vi "自由间隙.vi"(0 "曲线引用":refnum<vi>, 1 "自由间隙判定条件":cluster{"下限":dbl, "上限":dbl}, 3 "错误输入":errorcluster) -> (7 "曲线引用输出":refnum<vi>, 8 "OK？":bool, 10 "错误输出":errorcluster)   [LabVIEW 2018]
uses:
  Global_Variable/Global.vi
  Global_Variable/A180648.vi
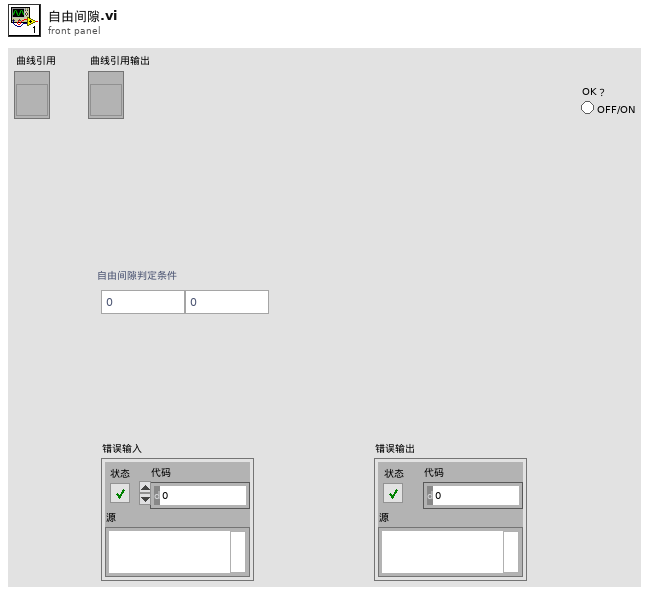
[diagram p1: front panel]
types:
  T1 = enum32{"空载", "功能", "力特性", "传感器特性", "电流特性", "振动NVH", "逆向空载", "完成"}
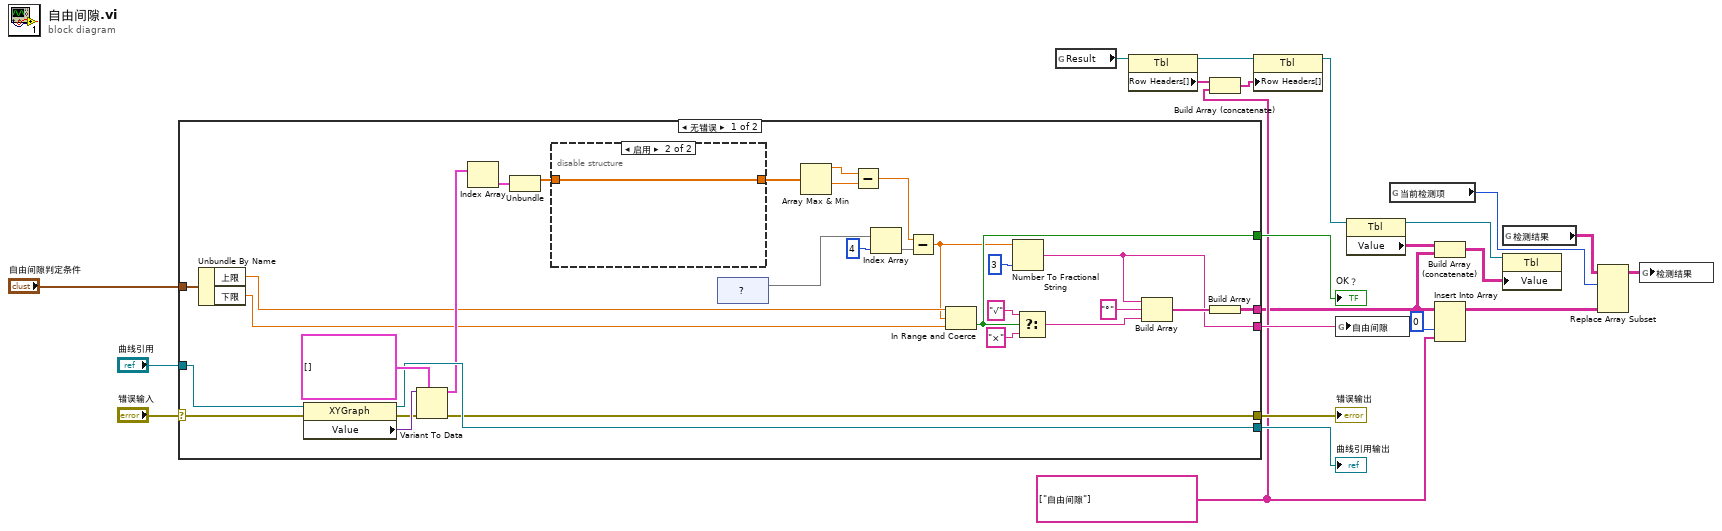
[diagram p0: block diagram]
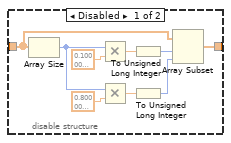
[diagram p2: hidden frame]
diagram:
  w7 = string[] ["自由间隙"] ("列首字符串[]")
  n1 = case shown="无错误" "错误输入" {
    selector: "错误输入" -> [w50 w64]
    tunnel: [w47 w64] -> w21
    tunnel: "曲线引用" -> [w46 w63]
    tunnel: [w49 w63] -> w19
    tunnel: [w33 _] -> w18
    tunnel: "自由间隙判定条件" -> [w36 _]
    tunnel: [w37 _] -> w1
    tunnel: [w25 _] -> w9
    frame No Error {
      n2 = Unbundle By Name(w36) -> ("上限"=w35:dbl, "下限"=w34:dbl)
      n3 = property class="XYGraph"(reference=w46, error in=w50) -> (reference out=w49:refnum<vi>, error out=w48:errorcluster, "Value"=w52:variant)
      n4 = Variant To Data(error in=w48, type=cluster{dbl[], dbl[]}[] [], Variant=w52) -> (data=w40:cluster{dbl[], dbl[]}[], error out=w47:errorcluster)
      n5 = Index Array(array=w40) -> (element=w39:cluster{dbl[], dbl[]})  [unwired: 1 in]
      n6 = Unbundle(w39) -> (w24:dbl[])  [unwired: 1 out]
      n7 = disable-structure shown="启用" {
        disable-tunnel: w24 -> [w54 w62]
        disable-tunnel: [w53 w62] -> w23
        frame Disabled {
          n8 = Array Size(array=w54) -> (size(s)=w57:i32)
          n9 = Multiply(x=w57, y=sgl 0.1) -> (x*y=w59:sgl)
          n10 = Multiply(x=w57, y=sgl 0.8) -> (x*y=w60:sgl)
          n11 = To Unsigned Long Integer(number=w59) -> (unsigned 32bit integer=w61:u32)
          n12 = To Unsigned Long Integer(number=w60) -> (unsigned 32bit integer=w58:u32)
          n13 = Array Subset(array=w54, index=w61, length=w58) -> (w53:dbl[])
        }
        frame Enabled {
        }
      }
      n14 = shared-variable "?"() -> (w29)  [unwired: 1 in, 1 out]
      n15 = Array Max & Min(array=w23) -> (max value=w32:dbl, min value=w31:dbl)  [unwired: 2 out]
      n16 = Subtract(x=w32, y=w31) -> (x-y=w30:dbl)
      n17 = Index Array(array=w29, index=4 ("索引")) -> (element=w27)
      n18 = Subtract(x=w30, y=w27) -> (x-y=w26:dbl)
      n19 = In Range and Coerce(upper limit=w35, x=w26, lower limit=w34) -> (In Range?=w33:bool)  [unwired: 1 out]
      n20 = Number To Fractional String(number=w26, precision (6)=i16 3 ("精度(6)")) -> (F-format string=w25:string)  [unwired: 2 in]
      n21 = Select(t="√" ("元素"), s=w33, f="×" ("元素")) -> (s? t:f=w41:string)
      n22 = Build Array(w25, "°" ("元素"), w41) -> (w38:string[])
      n23 = Build Array(w38) -> (w37:string[][])
    }
    frame Error {
    }
  }
  "错误输出" <- w21
  "曲线引用输出" <- w19
  "OK？" <- w18
  n24 = global read "Global.vi" "Result"() -> (w15:refnum<vi>)
  n25 = property class="Tbl"(reference=w15) -> (reference out=w14:refnum<vi>, "Row Headers[]"=w12:string[])  [unwired: 1 in, 1 out]
  n26 = Build Array (concatenate)(w12, w7) -> (w11:string[])
  n27 = property class="Tbl"(reference=w14, "Row Headers[]"=w11) -> (reference out=w13:refnum<vi>)  [unwired: 1 in, 1 out]
  n28 = global write "检测结果.vi" "自由间隙"(w9) -> ()
  n29 = property class="Tbl"(reference=w13) -> (reference out=w17:refnum<vi>, "Value"=w16:string[][])  [unwired: 1 in, 1 out]
  n30 = global read "A180648.vi" "当前检测项"() -> (w4:T1)
  n31 = Build Array (concatenate)(w16, w1) -> (w8:string[][])
  n32 = Insert Into Array(array=w1, index (col)=0 ("禁用的索引 (列)"), new element=w7) -> (w2:string[][])  [unwired: 1 in]
  n33 = global read "A180648.vi" "检测结果"() -> (w5:string[][][])
  n34 = property class="Tbl"(reference=w17, "Value"=w8) -> ()  [unwired: 1 in, 2 out]
  n35 = Replace Array Subset(array=w5, new element=w2, index (dim 0)=w4) -> (w3:string[][][])  [unwired: 2 in]
  n36 = global write "A180648.vi" "检测结果"(w3) -> ()
